vi "设定雇员信息.vi"(6 "职务":string, 8 "error in (no error)":errorcluster caption="错误输入（无错误）", 9 "年龄":u8, 10 "姓名":string, 11 "雇员 输入":refnum<class "雇员.lvclass"> caption="DNL_LabVIEW Object in") -> (0 "error out":errorcluster caption="错误输出", 3 "雇员 输出":refnum<class "雇员.lvclass"> caption="DNL_LabVIEW Object out")   [LabVIEW 2011, in "迭代器.lvlib" / "雇员.lvclass"]
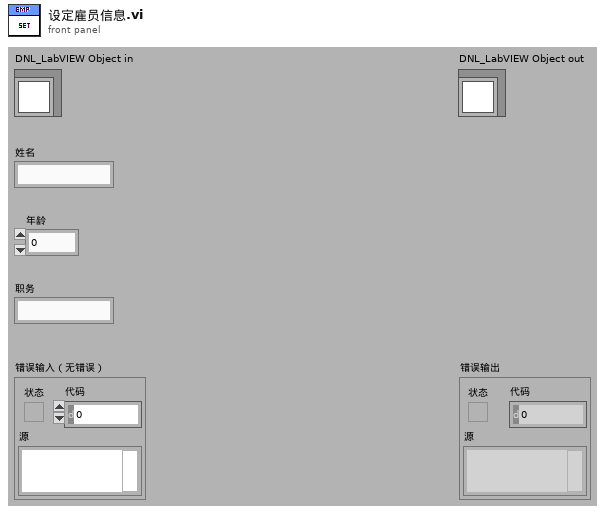
[diagram p1: front panel]
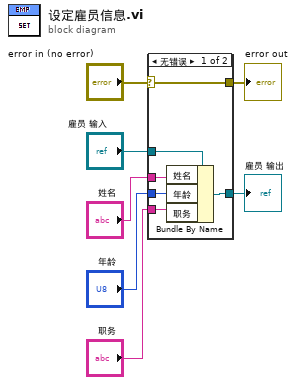
[diagram p0: block diagram]
diagram:
  n1 = case shown="无错误" "error in (no error)" {
    selector: "error in (no error)" -> [w13 w15]
    tunnel: [w13 w15] -> w6
    tunnel: [w11 w14] -> w4
    tunnel: "雇员 输入" -> [w12 w14]
    tunnel: "姓名" -> [w10 _]
    tunnel: "年龄" -> [w9 _]
    tunnel: "职务" -> [w8 _]
    frame No Error {
      n2 = Bundle By Name(cluster=w12, "姓名"=w10, "年龄"=w9, "职务"=w8) -> (w11:refnum<class "雇员.lvclass">)
    }
    frame Error {
    }
  }
  "error out" <- w6
  "雇员 输出" <- w4
